vi "Create DPID.vi"(8 "error in (no error)":errorcluster, 10 "DPID":T2, 11 "Section Ptr":T1 format="%.0x") -> (0 "error out":errorcluster, 3 "Parent Ref out":T1 format="%.0x")   [LabVIEW 2013, in "Diagnostics Addon Shared.lvlib"]
uses:
  Diagnostics Addon Shared.lvlib
  Exported DPID Parameters.ctl
  DPID Parameters.ctl
  DPID Periodic Rate.ctl
  <vilib>/NI Veristand/Custom Device API/Custom Device Item Ref.ctl
  GUID Lookup.vi
  <vilib>/NI Veristand/Custom Device API/Custom Device API.lvlib
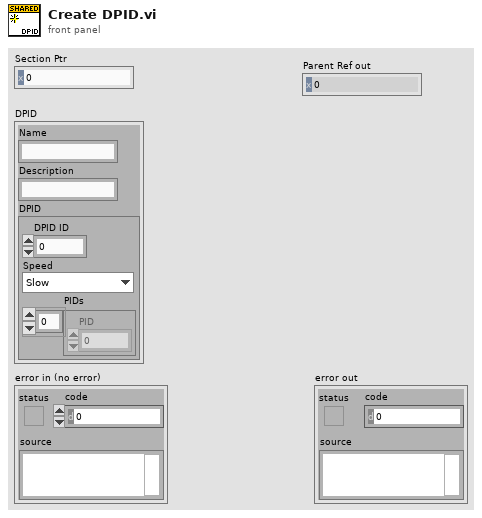
[diagram p1: front panel]
types:
  T1 = typedef "Custom Device API.lvlib/Custom Device Item Ref.ctl" = u64
  T2 = typedef "Diagnostics Addon Shared.lvlib/Exported DPID Parameters.ctl" = cluster{"Name":string, "Description":string, "DPID":T3}
  T3 = typedef "Diagnostics Addon Shared.lvlib/DPID Parameters.ctl" = cluster{"DPID ID":u8, "Speed":T4, "PIDs":u16[]}
  T4 = typedef "Diagnostics Addon Shared.lvlib/DPID Periodic Rate.ctl" = enum16{"Slow", "Medium", "Fast"}
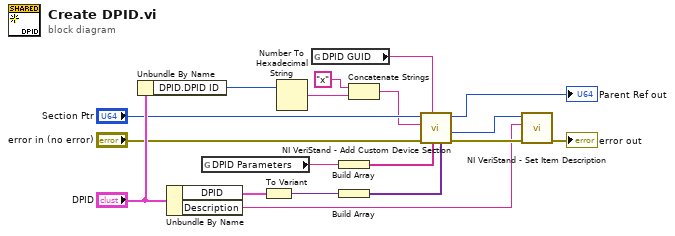
[diagram p0: block diagram]
diagram:
  n1 = Unbundle By Name("DPID") -> ("DPID.DPID ID"=w16:u8)
  n2 = Unbundle By Name("DPID") -> ("DPID"=w6:T3, "Description"=w2:string)
  n3 = global read "GUID Lookup.vi" "DPID Parameters"() -> (w12:string)
  n4 = To Variant(anything=w6) -> (Variant=w10:variant)
  n5 = Number To Hexadecimal String(2:w16) -> (0:w18:string)  [unwired: 1 in]
  n6 = global read "GUID Lookup.vi" "DPID GUID"() -> (w9:string)
  n7 = Build Array(w12) -> (w13:string[])
  n8 = Build Array(w10) -> (w11:variant[])
  n9 = Concatenate Strings("x" ("string"), w18) -> (w5:string)
  n10 = call <vilib>:"NI VeriStand - Add Custom Device Section.vi"("Property Values"=w11, "Property names"=w13, "GUID (Default Section)"=w9, "error in (no error)"="error in (no error)", "Section Name"=w5, "Parent Ref in"="Section Ptr") -> ("error out"=w14:errorcluster, "Section Ptr"=w3:T1, "Parent Ref out"=→"Parent Ref out":T1)  [unwired: 2 in, 1 out]
  n11 = call <vilib>:"NI VeriStand - Set Item Description.vi"("error in (no error)"=w14, "Description"=w2, "Item Ref in"=w3) -> ("error out"=→"error out":errorcluster)  [unwired: 6 in, 2 out]
